vi "啮合间隙判定.vi"(0 "曲线引用":refnum<vi>, 2 "曲线判定条件":cluster{"最大值":string, "最小值":string}, 3 "错误输入":errorcluster) -> (7 "曲线引用输出":refnum<vi>, 8 "判定结果":cluster{"合格？":bool, "判定结果":string[][]}, 10 "错误输出":errorcluster)   [LabVIEW 2018]
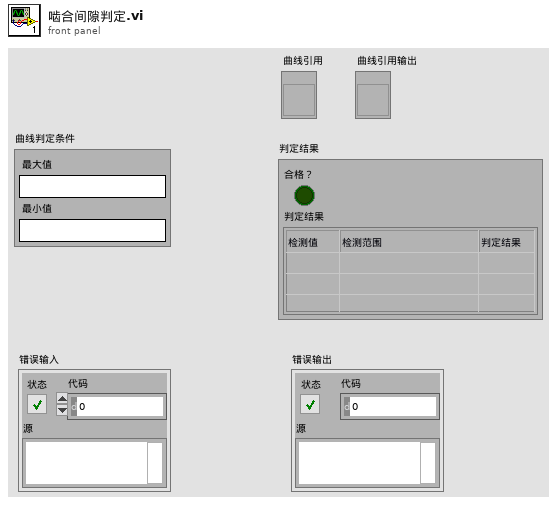
[diagram p1: front panel]
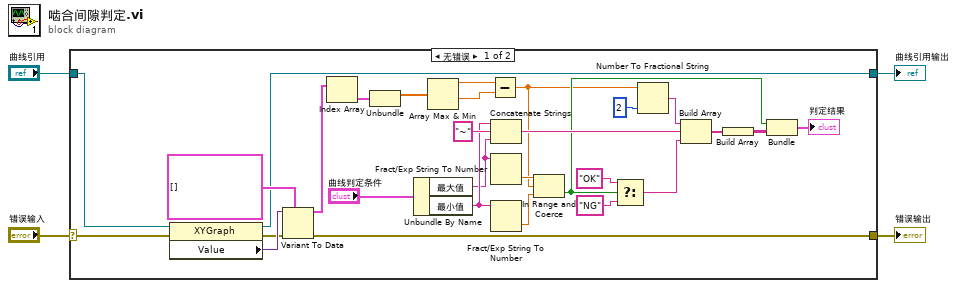
[diagram p0: block diagram]
diagram:
  n1 = case shown="无错误" "错误输入" {
    selector: "错误输入" -> [w31 w35]
    tunnel: [w25 w35] -> w3
    tunnel: "曲线引用" -> [w28 w34]
    tunnel: [w27 w34] -> w1
    frame No Error {
      n2 = property class="XYGraph"(reference=w28, error in=w31) -> (reference out=w27:refnum<vi>, error out=w26:errorcluster, "Value"=w33:variant)
      n3 = Variant To Data(error in=w26, type=cluster{dbl[], dbl[]}[] [], Variant=w33) -> (data=w24:cluster{dbl[], dbl[]}[], error out=w25:errorcluster)
      n4 = Index Array(array=w24) -> (element=w30:cluster{dbl[], dbl[]})  [unwired: 1 in]
      n5 = Unbundle(w30) -> (w23:dbl[])  [unwired: 1 out]
      n6 = Unbundle By Name("曲线判定条件") -> ("最大值"=w5:string, "最小值"=w6:string)
      n7 = Array Max & Min(array=w23) -> (max value=w21:dbl, min value=w20:dbl)  [unwired: 2 out]
      n8 = Subtract(x=w21, y=w20) -> (x-y=w7:dbl)
      n9 = Concatenate Strings(w6, "~" ("字符串"), w5) -> (w11:string)
      n10 = Fract/Exp String To Number(string=w5) -> (number=w19:dbl)  [unwired: 3 in, 1 out]
      n11 = Fract/Exp String To Number(string=w6) -> (number=w18:dbl)  [unwired: 3 in, 1 out]
      n12 = In Range and Coerce(upper limit=w19, x=w7, lower limit=w18) -> (In Range?=w9:bool)  [unwired: 1 out]
      n13 = Select(t="OK", s=w9, f="NG") -> (s? t:f=w13:string)
      n14 = Number To Fractional String(number=w7, precision (6)=i16 2 ("精度(6)")) -> (F-format string=w16:string)  [unwired: 2 in]
      n15 = Build Array(w16, w11, w13) -> (w29:string[])
      n16 = Build Array(w29) -> (w10:string[][])
      n17 = Bundle(w9, w10) -> (→"判定结果":cluster{bool, string[][]})  [unwired: 1 in]
    }
    frame Error {
    }
  }
  "错误输出" <- w3
  "曲线引用输出" <- w1
